vi "STM32.MISC.vi"(7 "Error In":errorcluster caption="错误输入", 9 "CMD":enum16{"Version", "List SDcard Files", "RESET"}(ring), 10 "VISA资源输入":refnum<visa-resource-name>) -> (0 "Error Out":errorcluster caption="错误输出", 1 "附加数据":string, 2 "返回":string)   [LabVIEW 2012, in "Lib_UEL.ATE.lvlib" / "STM32-CoreBD.lvlib"]
uses:
  STM32-CoreBD.lvlib
panel:
  # "Version History\nV01,2014-4-14, 初始版本."
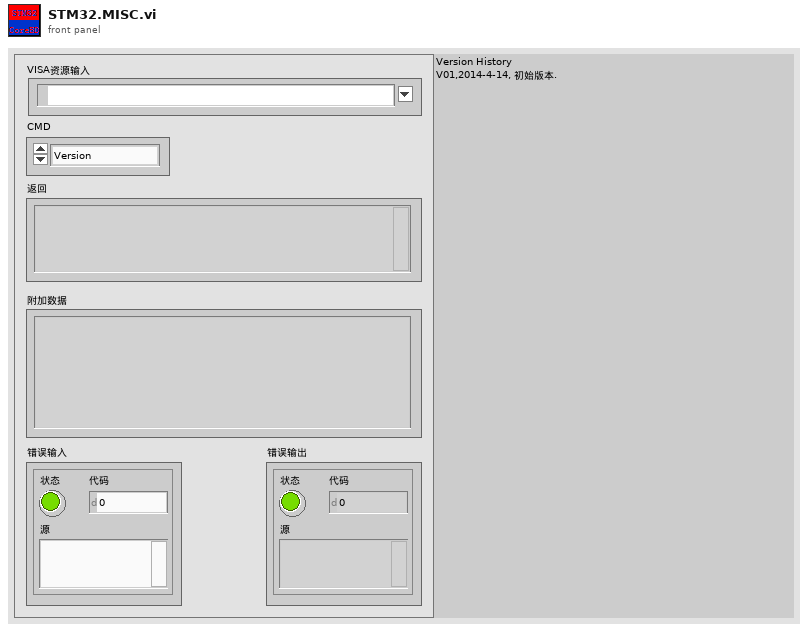
[diagram p1: front panel]
types:
  T1 = enum16{"Version", "SD Card Status", "WAV filelist", "RESET"}
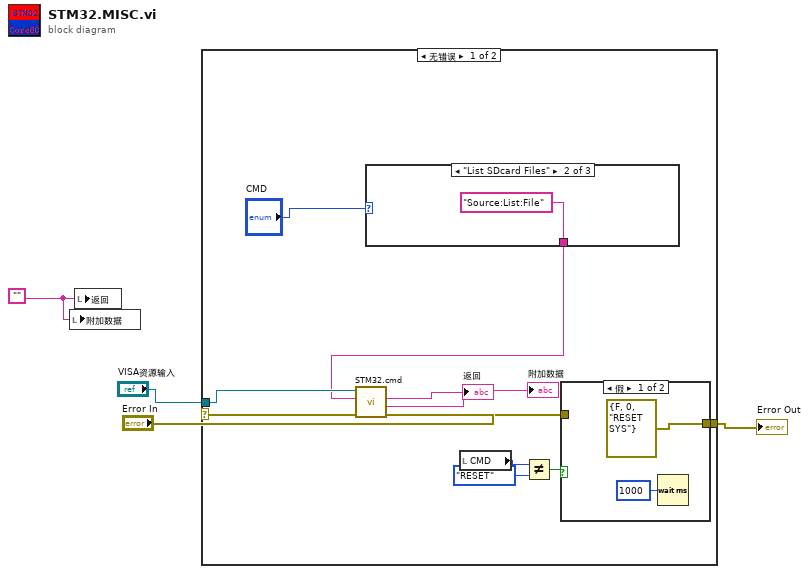
[diagram p0: block diagram]
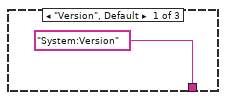
[diagram p3: hidden frame]
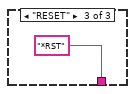
[diagram p4: hidden frame]
diagram:
  w1 = ""
  n1 = local write "附加数据"(w1) -> ()
  n2 = local write "返回"(w1) -> ()
  n3 = case shown="无错误" "Error In" {
    selector: "Error In" -> [w13 w22]
    tunnel: [w6 w22] -> w4
    tunnel: "VISA资源输入" -> [w14 _]
    frame No Error {
      n4 = case shown="\"List SDcard Files\"" "CMD" {
        tunnel: ["System:Version" ("字符串") "Source:List:File" ("字符串") "*RST" ("字符串")] -> w5
        frame "Version", Default {
        }
        frame "List SDcard Files" {
        }
        frame "RESET" {
        }
      }
      n5 = call "STM32.cmd.vi"("Error In"=w13, "命令"=w5, "VISA资源输入"=w14) -> ("Error Out"=w7:errorcluster, "附加数据"=→"附加数据":string, "返回"=→"返回":string)  [unwired: 5 in, 1 out]
      n6 = local read "CMD"() -> (w10:enum16{"Version", "List SDcard Files", "RESET"})
      n7 = Not Equal?(x=w10, y=T1."RESET") -> (x != y?=w8:bool)
      n8 = case shown="假" w8 {
        tunnel: w7 -> [_ w18]
        tunnel: [errorcluster {"status"=FALSE, "code"=0, "source"="RESET SYS"} ("Error Out") w18] -> w6
        frame False {
          n9 = Wait (ms)(milliseconds to wait=u32 1000 ("等待时间（毫秒）")) -> ()  [unwired: 1 out]
        }
        frame True {
        }
      }
    }
    frame Error {
    }
  }
  "Error Out" <- w4
